vi "Get Stream State.vi"(8 "error in (no error)":errorcluster, 10 "stream index":i32, 11 "refnum in":refnum<k20>) -> (0 "error out":errorcluster, 2 "stream state":T1, 3 "refnum out":refnum<k20>)   [LabVIEW 2015, in "niInstr Streaming v1 Host.lvlib"]
doc: "Provides access to the current reported stream state from the FPGA.\n\n<B>Input Parameters</B>\n\n<B>error in (no error)</B> 'error in' can accept error information wired from VIs previously called. Use this information to decide if any functionality should be bypassed in the event of errors from other VIs.\n\nRight-click the 'error in' control on the front panel and select 'Explain Error' or 'Explain Warning' from the shortcut menu for more information about the error.\n\n<B>stream index</B> Selects which stream index this VI will interface to. This is the index number at the end of the host interface controls (0..7).\n\n<B>refnum in</B> Wire in the session obtained from Open FPGA Reference.\n\n<B>Output Parameters</B>\n\n<B>error out</B> contains error information. This output provides standard error out functionality.\n\n<B>refnum out</B> Copy of refnum in"
uses:
  <instrlib>/_niInstr/Streaming/v1/Host/niInstr Streaming v1 Host.lvlib
  <instrlib>/_niInstr/Streaming/v1/Common/Stream State.ctl
  <instrlib>/_niInstr/Streaming/v1/Host/Public/Stream Host Interface.ctl
  <vilib>/Utility/error.llb/Error Cluster From Error Code.vi
  <vilib>/rvi/errors/niLvFpgaAdjustHostInterfaceError.vi
  <vilib>/ErrorRing/Error Ring.xnode
  <vilib>/rvi/interface/nirviReadWriteControl/nirviReadWriteControl.xnode
  <vilib>/rvi/interface/Simulation/niFpgaSimulationCallBeginRW.vi
  NiFpgaLv.dll
  <instrlib>/_niInstr/Streaming/v1/Common/niInstr Streaming v1 Common.lvlib
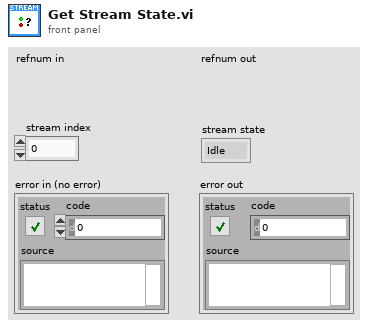
[diagram p1: front panel]
types:
  T1 = typedef "niInstr Streaming v1 Common.lvlib/Stream State.ctl" = enum8{"Idle", "Finite Transfer", "Continuous", "Done", "Error", "Not Ready", "Cancel"}
  T2 = typedef "niInstr Streaming v1 Host.lvlib/Stream Host Interface.ctl" = refnum<k20>
  T3 = enum8{"Idle", "Finite Transfer", "Continuous", "Done", "Error", "Not Ready", "Cancel"}
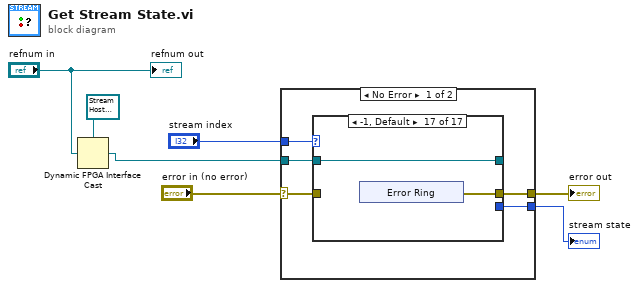
[diagram p0: block diagram]
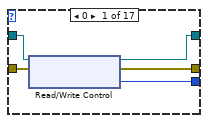
[diagram p2: hidden frame]
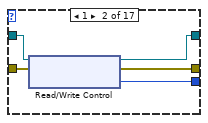
[diagram p3: hidden frame]
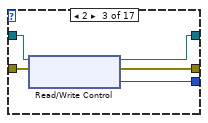
[diagram p4: hidden frame]
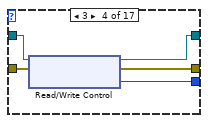
[diagram p5: hidden frame]
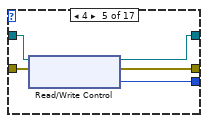
[diagram p6: hidden frame]
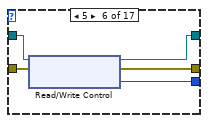
[diagram p7: hidden frame]
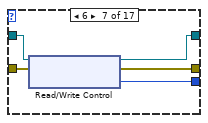
[diagram p8: hidden frame]
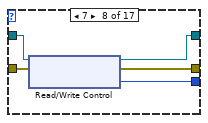
[diagram p9: hidden frame]
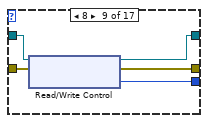
[diagram p10: hidden frame]
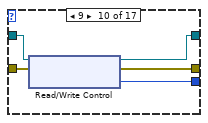
[diagram p11: hidden frame]
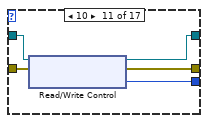
[diagram p12: hidden frame]
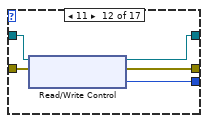
[diagram p13: hidden frame]
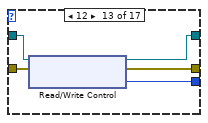
[diagram p14: hidden frame]
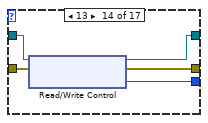
[diagram p15: hidden frame]
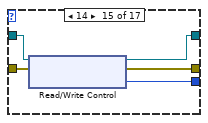
[diagram p16: hidden frame]
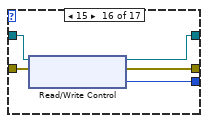
[diagram p17: hidden frame]
diagram:
  n1 = Dynamic FPGA Interface Cast(Session In=T2 refnum ("Refnum in"), Type="refnum in") -> (Session Out=w2:T2)
  n2 = case shown="No Error" "error in (no error)" {
    selector: "error in (no error)" -> [w8 w99]
    tunnel: [w12 _] -> w7
    tunnel: "stream index" -> [w11 _]
    tunnel: [w10 w99] -> w5
    tunnel: w2 -> [w9 _]
    frame No Error {
      n3 = case shown="-1, Default" w11 {
        tunnel: w8 -> [w17 w22 w27 w32 w37 w42 w47 w52 w57 w62 w67 w72 w77 w82 w87 w92 _]
        tunnel: [w16 w21 w26 w31 w36 w41 w46 w51 w56 w61 w66 w71 w76 w81 w86 w91 w94] -> _
        tunnel: [w15 w20 w25 w30 w35 w40 w45 w50 w55 w60 w65 w70 w75 w80 w85 w90 w93] -> w10
        tunnel: w9 -> [w14 w19 w24 w29 w34 w39 w44 w49 w54 w59 w64 w69 w74 w79 w84 w89 w94]
        tunnel: [w13 w18 w23 w28 w33 w38 w43 w48 w53 w58 w63 w68 w73 w78 w83 w88 _] -> w12
        frame 0 {
          n4 = xnode "Read/Write Control"("FPGA VI Reference In"=w14, "error in"=w17) -> ("FPGA VI Reference Out"=w16:T2, "error out"=w15:errorcluster, "stream.state 0"=w13:T3)
        }
        frame 1 {
          n5 = xnode "Read/Write Control"("FPGA VI Reference In"=w19, "error in"=w22) -> ("FPGA VI Reference Out"=w21:T2, "error out"=w20:errorcluster, "stream.state 1"=w18:T3)
        }
        frame 2 {
          n6 = xnode "Read/Write Control"("FPGA VI Reference In"=w24, "error in"=w27) -> ("FPGA VI Reference Out"=w26:T2, "error out"=w25:errorcluster, "stream.state 2"=w23:T3)
        }
        frame 3 {
          n7 = xnode "Read/Write Control"("FPGA VI Reference In"=w29, "error in"=w32) -> ("FPGA VI Reference Out"=w31:T2, "error out"=w30:errorcluster, "stream.state 3"=w28:T3)
        }
        frame 4 {
          n8 = xnode "Read/Write Control"("FPGA VI Reference In"=w34, "error in"=w37) -> ("FPGA VI Reference Out"=w36:T2, "error out"=w35:errorcluster, "stream.state 4"=w33:T3)
        }
        frame 5 {
          n9 = xnode "Read/Write Control"("FPGA VI Reference In"=w39, "error in"=w42) -> ("FPGA VI Reference Out"=w41:T2, "error out"=w40:errorcluster, "stream.state 5"=w38:T3)
        }
        frame 6 {
          n10 = xnode "Read/Write Control"("FPGA VI Reference In"=w44, "error in"=w47) -> ("FPGA VI Reference Out"=w46:T2, "error out"=w45:errorcluster, "stream.state 6"=w43:T3)
        }
        frame 7 {
          n11 = xnode "Read/Write Control"("FPGA VI Reference In"=w49, "error in"=w52) -> ("FPGA VI Reference Out"=w51:T2, "error out"=w50:errorcluster, "stream.state 7"=w48:T3)
        }
        frame 8 {
          n12 = xnode "Read/Write Control"("FPGA VI Reference In"=w54, "error in"=w57) -> ("FPGA VI Reference Out"=w56:T2, "error out"=w55:errorcluster, "stream.state 8"=w53:T3)
        }
        frame 9 {
          n13 = xnode "Read/Write Control"("FPGA VI Reference In"=w59, "error in"=w62) -> ("FPGA VI Reference Out"=w61:T2, "error out"=w60:errorcluster, "stream.state 9"=w58:T3)
        }
        frame 10 {
          n14 = xnode "Read/Write Control"("FPGA VI Reference In"=w64, "error in"=w67) -> ("FPGA VI Reference Out"=w66:T2, "error out"=w65:errorcluster, "stream.state 10"=w63:T3)
        }
        frame 11 {
          n15 = xnode "Read/Write Control"("FPGA VI Reference In"=w69, "error in"=w72) -> ("FPGA VI Reference Out"=w71:T2, "error out"=w70:errorcluster, "stream.state 11"=w68:T3)
        }
        frame 12 {
          n16 = xnode "Read/Write Control"("FPGA VI Reference In"=w74, "error in"=w77) -> ("FPGA VI Reference Out"=w76:T2, "error out"=w75:errorcluster, "stream.state 12"=w73:T3)
        }
        frame 13 {
          n17 = xnode "Read/Write Control"("FPGA VI Reference In"=w79, "error in"=w82) -> ("FPGA VI Reference Out"=w81:T2, "error out"=w80:errorcluster, "stream.state 13"=w78:T3)
        }
        frame 14 {
          n18 = xnode "Read/Write Control"("FPGA VI Reference In"=w84, "error in"=w87) -> ("FPGA VI Reference Out"=w86:T2, "error out"=w85:errorcluster, "stream.state 14"=w83:T3)
        }
        frame 15 {
          n19 = xnode "Read/Write Control"("FPGA VI Reference In"=w89, "error in"=w92) -> ("FPGA VI Reference Out"=w91:T2, "error out"=w90:errorcluster, "stream.state 15"=w88:T3)
        }
        frame -1, Default {
          n20 = xnode "Error Ring"() -> ("error out"=w93:errorcluster)
        }
      }
    }
    frame Error {
    }
  }
  "stream state" <- w7
  "error out" <- w5
  "refnum out" <- "refnum in"
